vi "timekeeper sync time.vi"(0 "Slave time":fxp<+,64,64>, 1 "Master time":fxp<+,64,64>) -> ()   [LabVIEW 2011, in "EPS_Timekeeper.lvlib"]
uses:
  <vilib>/addons/Electrical Power/Example Support/PMU/Time Keeper/EPS_Timekeeper.lvlib
  <vilib>/addons/Electrical Power/Example Support/PMU/Time Keeper/timekeeper timereference timestamp (g).vi
  <vilib>/addons/Electrical Power/Example Support/PMU/Time Keeper/timekeeper timereference time (g).vi
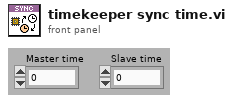
[diagram p1: front panel]
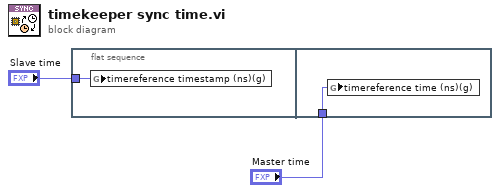
[diagram p0: block diagram]
diagram:
  n1 = flat-sequence {
    tunnel: "Slave time" -> [w3]
    tunnel: "Master time" -> [w4]
    frame #0 {
      n2 = global write "timekeeper timereference timestamp (g).vi" "timereference timestamp (ns)(g)"(w3) -> ()
    }
    frame #1 {
      n3 = global write "timekeeper timereference time (g).vi" "timereference time (ns)(g)"(w4) -> ()
    }
  }
